vi "ShootingPID.vi"() -> (3 "Output":dbl)   [LabVIEW 2016]
uses:
  Robot Global Data.vi
  <vilib>/addons/control/pid/pid.llb/PID (DBL).vi
  <vilib>/addons/control/pid/NI_PID_pid.lvlib
panel:
  out "Encoder":dbl(graph)
  in  "Setpoint":dbl format="%#_13g"
  in  "PID gains":T1={"proportional gain (Kc)"=0.019, "integral time (Ti, min)"=0.0, "derivative time (Td, min)"=0.0} {"derivative time (Td, min)" format="%.3f"; "integral time (Ti, min)" format="%.3f"; "proportional gain (Kc)" format="%.3f"}
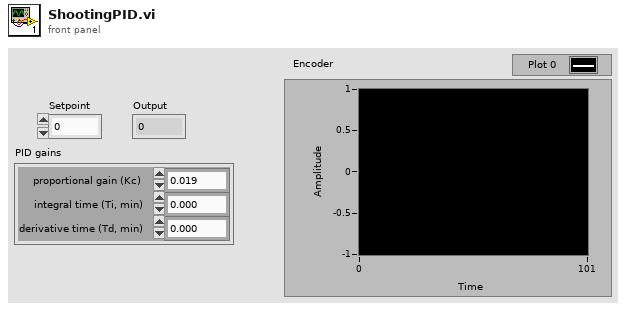
[diagram p1: front panel]
types:
  T1 = cluster{"proportional gain (Kc)":dbl, "integral time (Ti, min)":dbl, "derivative time (Td, min)":dbl}
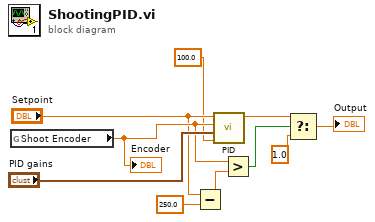
[diagram p0: block diagram]
diagram:
  n1 = global read "Robot Global Data.vi" "Shoot Encoder"() -> (w6:dbl)
  "Encoder" <- w6
  n2 = Subtract(x="Setpoint", y=250.0) -> (x-y=w4:dbl)
  n3 = call-poly <vilib>:"PID.vi"("dt (s)"=100.0, "PID gains"="PID gains", "process variable"=w6, "setpoint"="Setpoint") -> ("output"=w8:dbl)  [unwired: 6 in, 1 out]
  n4 = Greater?(x=w6, y=w4) -> (0:w7:bool)
  n5 = Select(t=w8, s=w7, f=1.0) -> (s? t:f=→"Output":dbl)
